vi "Check status.vi"(8 "Error In":errorcluster, 11 "VISA resource in":refnum<visa-resource-name>) -> (0 "Error Out":errorcluster, 2 "Is Done?":bool, 3 "VISA resource out":refnum<visa-resource-name>, 4 "read buffer":string)   [LabVIEW 2014, in "Motor manager.lvlib"]
uses:
  Motor manager.lvlib
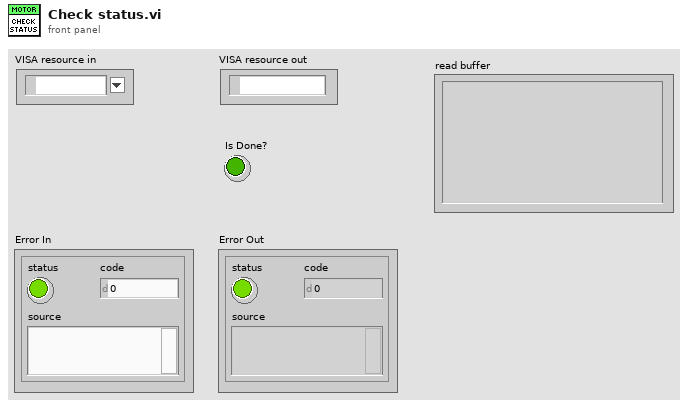
[diagram p1: front panel]
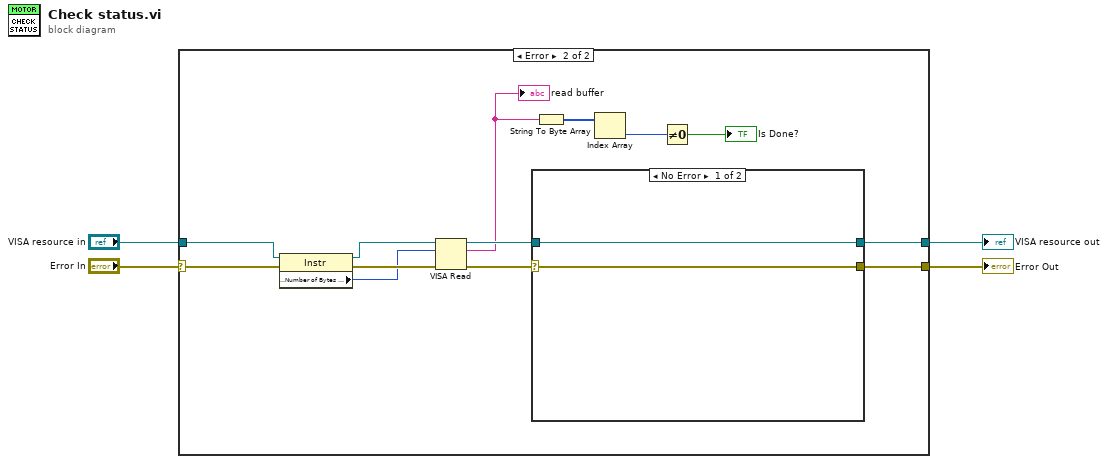
[diagram p0: block diagram]
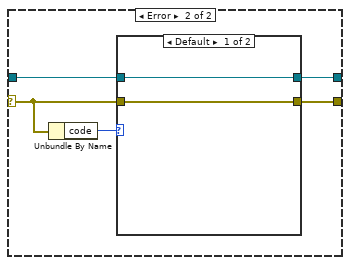
[diagram p3: hidden frame]
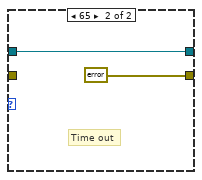
[diagram p4: hidden frame]
diagram:
  n1 = case shown="Error" "Error In" {
    selector: "Error In" -> [w6 w19]
    tunnel: "VISA resource in" -> [w5 w16]
    tunnel: [w6 w13] -> w2
    tunnel: [w5 w11] -> w1
    frame No Error {
    }
    frame Error {
      n2 = property class="Instr"(reference=w16, error in=w19) -> (reference out=w17:refnum<visa-resource-name>, error out=w18:errorcluster, "Serial Settings:Number of Bytes at Serial Port"=w15:u32)
      n3 = VISA Read(VISA resource name=w17, byte count=w15, error in (no error)=w18) -> (VISA resource name out=w12:refnum<visa-resource-name>, read buffer=w10:string, error out=w14:errorcluster)  [unwired: 1 out]
      "read buffer" <- w10
      n4 = case shown="No Error" w14 {
        selector: w14 -> [w21 w25]
        tunnel: [w21 w24] -> w13
        tunnel: w12 -> [w20 w23]
        tunnel: [w20 w22] -> w11
        frame No Error {
        }
        frame Error {
          n5 = Unbundle By Name(w25) -> ("code"=w26:i32)
          n6 = case shown="Default" w26 {
            tunnel: w25 -> [w28 _]
            tunnel: [w28 errorcluster {"status"=FALSE, "code"=0, "source"=""} ("error IO")] -> w24
            tunnel: [w27 w29] -> w22
            tunnel: w23 -> [w27 w29]
            frame Default {
            }
            frame 65 {
              # "Time out"
            }
          }
        }
      }
      n7 = String To Byte Array(string=w10) -> (unsigned byte array=w8:u8[])
      n8 = Index Array(array=w8) -> (element=w7:u8)  [unwired: 1 in]
      n9 = Not Equal To 0?(x=w7) -> (x != 0?=→"Is Done?":bool)
    }
  }
  "VISA resource out" <- w1
  "Error Out" <- w2
